vi "SetBKValue.vi"(7 "Command":T1=enum."MaxVoltage", 8 "error in (no error)":errorcluster, 9 "Value":string, 10 "Channel":string, 11 "Connection In":refnum<k5>) -> (0 "error out":errorcluster, 3 "Connection Out":refnum<k5>)   [LabVIEW 2020]
uses:
  CommandTypeDef.ctl
panel:
  out "Sent Message":string
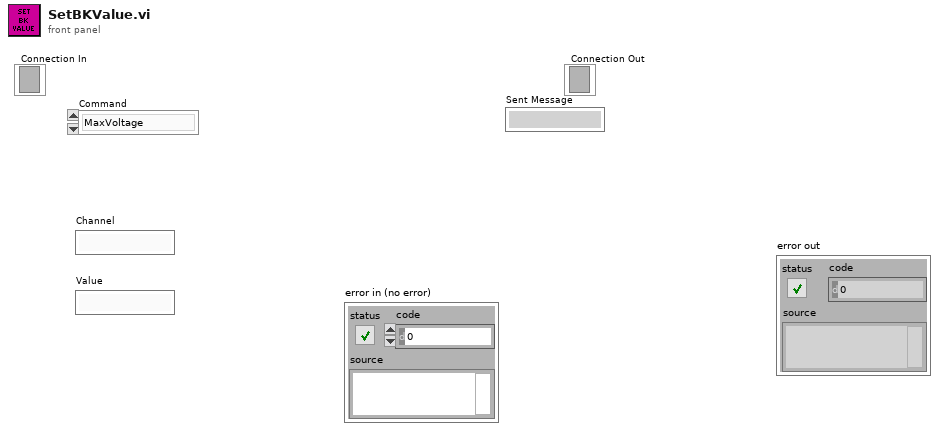
[diagram p1: front panel]
types:
  T1 = typedef "CommandTypeDef.ctl" = enum16{"Current", "MaxVoltage", "SlewRate", "EnableOutput", "Reset", "CurrentVoltage", "MaxCurrent"}
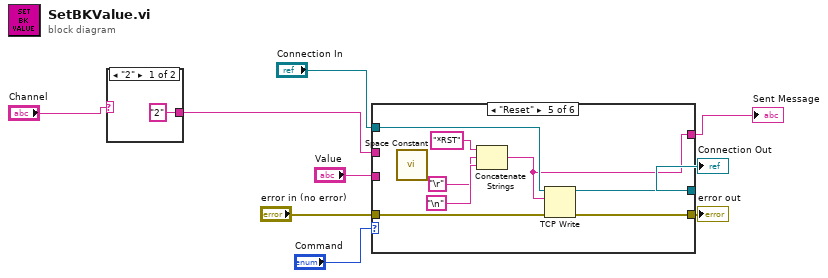
[diagram p0: block diagram]
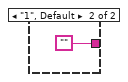
[diagram p2: hidden frame]
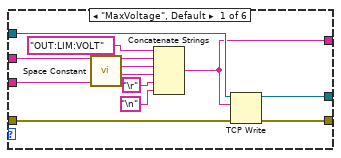
[diagram p3: hidden frame]
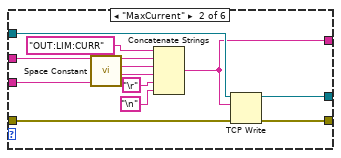
[diagram p4: hidden frame]
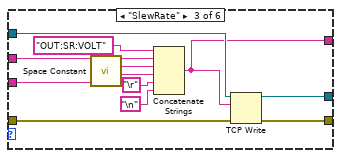
[diagram p5: hidden frame]
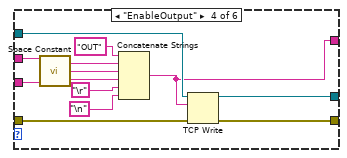
[diagram p6: hidden frame]
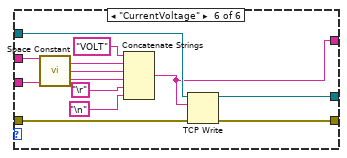
[diagram p7: hidden frame]
diagram:
  n1 = case shown="\"2\"" "Channel" {
    tunnel: ["2" ""] -> w1
    frame "2" {
    }
    frame "1", Default {
    }
  }
  n2 = case shown="\"Reset\"" "Command" {
    tunnel: "Connection In" -> [w18 w29 w40 w51 w60 w72]
    tunnel: [w17 w28 w35 w46 w57 w71] -> w7
    tunnel: [w16 w27 w36 w47 w58 w70] -> w6
    tunnel: "error in (no error)" -> [w15 w26 w37 w48 w59 w69]
    tunnel: w1 -> [w13 w24 w39 w50 _ w67]
    tunnel: "Value" -> [w14 w25 w38 w49 _ w65]
    tunnel: [w12 w23 w34 w45 w56 w64] -> w3
    frame "MaxVoltage", Default {
      n3 = call "Space Constant.vi"() -> ("String"=w19:string)
      n4 = Concatenate Strings("OUT:LIM:VOLT" ("data in"), w13, w19, w14, "\r", "\n") -> (w12:string)
      n5 = TCP Write(connection ID=w18, data in=w12, error in (no error)=w15) -> (connection ID out=w17:refnum<k5>, error out=w16:errorcluster)  [unwired: 1 in, 1 out]
    }
    frame "MaxCurrent" {
      n6 = call "Space Constant.vi"() -> ("String"=w30:string)
      n7 = Concatenate Strings("OUT:LIM:CURR" ("data in"), w24, w30, w25, "\r", "\n") -> (w23:string)
      n8 = TCP Write(connection ID=w29, data in=w23, error in (no error)=w26) -> (connection ID out=w28:refnum<k5>, error out=w27:errorcluster)  [unwired: 1 in, 1 out]
    }
    frame "SlewRate" {
      n9 = call "Space Constant.vi"() -> ("String"=w41:string)
      n10 = Concatenate Strings("OUT:SR:VOLT" ("data in"), w39, w41, w38, "\r", "\n") -> (w34:string)
      n11 = TCP Write(connection ID=w40, data in=w34, error in (no error)=w37) -> (connection ID out=w35:refnum<k5>, error out=w36:errorcluster)  [unwired: 1 in, 1 out]
    }
    frame "EnableOutput" {
      n12 = call "Space Constant.vi"() -> ("String"=w52:string)
      n13 = Concatenate Strings("OUT" ("data in"), w50, w52, w49, "\r", "\n") -> (w45:string)
      n14 = TCP Write(connection ID=w51, data in=w45, error in (no error)=w48) -> (connection ID out=w46:refnum<k5>, error out=w47:errorcluster)  [unwired: 1 in, 1 out]
    }
    frame "Reset" {
      n15 = call "Space Constant.vi"() -> ()  [unwired: 1 out]
      n16 = Concatenate Strings("*RST" ("data in"), "\r", "\n") -> (w56:string)
      n17 = TCP Write(connection ID=w60, data in=w56, error in (no error)=w59) -> (connection ID out=w57:refnum<k5>, error out=w58:errorcluster)  [unwired: 1 in, 1 out]
    }
    frame "CurrentVoltage" {
      n18 = call "Space Constant.vi"() -> ("String"=w66:string)
      n19 = Concatenate Strings("VOLT" ("data in"), w67, w66, w65, "\r", "\n") -> (w64:string)
      n20 = TCP Write(connection ID=w72, data in=w64, error in (no error)=w69) -> (connection ID out=w71:refnum<k5>, error out=w70:errorcluster)  [unwired: 1 in, 1 out]
    }
  }
  "Connection Out" <- w7
  "error out" <- w6
  "Sent Message" <- w3
